vi "Set Data Ready Event.vi"(8 "error in (no error)":errorcluster, 11 "dataevent":u32) -> (0 "error out":errorcluster, 3 "dataevent out":u32)   [LabVIEW 2021, in "vmmso.lvlib"]
doc: "DLL_API void WINAPI SetDataReadyEvent(HANDLE dataevent);"
uses:
  vmmso.lvlib
  vmmso.dll
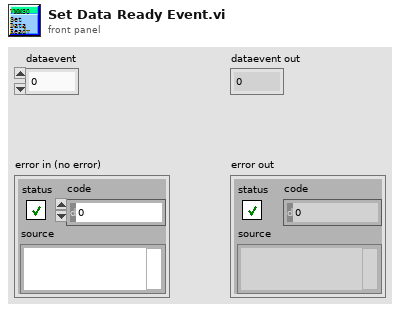
[diagram p1: front panel]
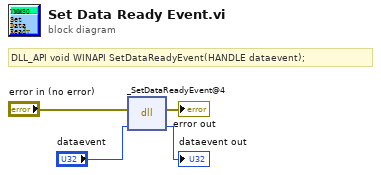
[diagram p0: block diagram]
diagram:
  # "DLL_API void WINAPI SetDataReadyEvent(HANDLE dataevent);"
  n1 = dll-call lib="O:/MSO/library/demo-Labview/vmmso/vmmso.*" fn="_SetDataReadyEvent@4"(error in="error in (no error)", "dataevent"="dataevent") -> (error out=→"error out":errorcluster, "dataevent"=→"dataevent out":u32)  [unwired: 3 in, 1 out]
